vi "Dashboard Main.vi"() -> ()   [LabVIEW 2017]
uses:
  <vilib>/Rock Robotics/WPI/DriverStation/WPI_DriverStationAllianceInfo.ctl
  <vilib>/Utility/miscctls.llb/LVRowAndColumnTypeDef.ctl
  <vilib>/event_ctls.llb/eventvkey.ctl
  <vilib>/Rock Robotics/Network Tables/NT Read Numeric Array.vi
  <vilib>/Rock Robotics/WPI/Dashboard/WPI_DashboardLogging Global.vi
  <vilib>/Rock Robotics/Network Tables/NT Write Numeric Array.vi
  <vilib>/Rock Robotics/Network Tables/NT Write Boolean.vi
panel:
  in  "Camera Settings Right":T1={"Frame Rate"=30, "Compression"=30, "Size"=1, "DB Camera Config"=FALSE} {"Frame Rate" scale=1.0..30.0; "Compression" scale=100.0..-1.0; "Size" items=["640x480", "320x240", "160x120"]}
  in  "Camera Name Right":string(combo)="No Camera Selection"
  out "Camera Info":cluster{"Mbps LED":bool, "Mbps":dbl, "fps":dbl} {"fps" format="%#.1g"; "Mbps" format="%#.1g"}
  in  "Camera Settings":T1={"Frame Rate"=30, "Compression"=30, "Size"=1, "DB Camera Config"=FALSE} {"Frame Rate" scale=1.0..30.0; "Compression" scale=100.0..-1.0; "Size" items=["640x480", "320x240", "160x120"]}
  in  "TCP":refnum<k5>
  in  "Rec Mode":enum32{"Stop", "Record", "Playback"}(radio)
  out "Robot IP":string
  out "Image Message":string="Timeout in Camera Communications"
  in  "Dashboard Tab":T2(tab)=enum."Custom"
  in  "Select Auto":string(combo)="Select Autonomous ..."
  out "NT Connection":bool
  out "MotorChart R":cluster{"Numeric":dbl, "Numeric":dbl}(graph)
  out "MotorChart L":cluster{"Numeric":dbl, "Numeric":dbl}(graph)
  out "MotorSliders R":cluster{"MotorSlide1":dbl, "MotorSlide2":dbl} {"MotorSlide2" scale=-1.0..1.0 scale format="%#_2e"; "MotorSlide1" scale=-1.0..1.0 scale format="%#_2e"}
  out "MotorSliders L":cluster{"MotorSlide1":dbl, "MotorSlide2":dbl} {"MotorSlide2" scale=-1.0..1.0 scale format="%#_2e"; "MotorSlide1" scale=-1.0..1.0 scale format="%#_2e"}
  out "Gyro":dbl(knob) scale=0.0..360.0
  out "JS1 Z":dbl(slide) scale=-1.0..1.0 scale format="%#_2e"
  out "JS1 Graph":cluster{"X":dbl, "Y":dbl}[](graph)
  out "JS1 Buttons":T3
  out "JS2 Z":dbl(slide) scale=-1.0..1.0 scale format="%#_2e"
  out "JS2 Graph":cluster{"X":dbl, "Y":dbl}[](graph)
  out "JS2 Buttons":T3
  out "Mode":T4(ring)=enum."Auto Disabled"
  out "Camera Image Right":T5(plugin-control)
  in  "DB/String 9":string
  in  "DB/String 8":string
  in  "DB/String 7":string
  in  "DB/String 6":string
  in  "DB/String 5":string
  in  "DB/String 4":string
  in  "DB/String 3":string
  in  "DB/String 2":string
  in  "DB/String 1":string
  in  "DB/String 0":string
  in  "DB/Slider 0":dbl(slide) scale=0.0..5.0
  in  "DB/Slider 1":dbl(slide) scale=0.0..5.0
  in  "DB/Slider 2":dbl(slide) scale=0.0..5.0
  in  "DB/Slider 3":dbl(slide) scale=0.0..5.0
  out "DB/LED 3":bool
  out "DB/LED 2":bool
  out "DB/LED 1":bool
  out "DB/LED 0":bool
  in  "DB/Button 3":bool
  in  "DB/Button 2":bool
  in  "DB/Button 1":bool
  in  "DB/Button 0":bool caption="New Name"
  in  "Delay":dbl
  in  "NotPurePursuit":bool
  in  "Battery Number":string
  out "Opponent Left Switch":bool
  out "Opponent Right Switch":bool
  out "Center Left Scale":bool
  out "Center Right Scale":bool
  out "Our Left Team Switch":bool
  out "Our Right Team Switch":bool
  in  "Position":u32=3
  in  "Routine":u32
  in  "SwitchOtherClose":u32
  in  "SwitchOtherNotClose":u32
  in  "ScaleOtherClose":u32
  in  "ScaleOtherNotClose":u32
  in  "Test Slider":dbl(slide) scale=0.0..100.0 scale format="%#_3g"
  in  "On/Off":bool caption="Solenoid"
  in  "Test Name":u16(ring) items=["Select the test to run..."]
  in  "Test Tree":string(tree)
  in  "Motor":cluster{"Value":dbl, "Enable":bool} {"Value" scale=-1.0..1.0 scale format="%#_3g"}
  out "Progress":T6 {"Test Progress" scale=0.0..100.0}
  in  "Rev/Fwd":cluster{"Forward":bool, "Reverse":bool}
  in  "Test Ring":u16(ring) items=["Monochrome", "Color"]
  out "Cmd Status":string
  in  "Execute Command":bool
  in  "Command Params":string[][](table)
  in  "Command Selection":i32(listbox)
  in  "CheckList":i32(listbox)
  out "Tree":string(tree)
  out "Camera Image":T5(plugin-control)
  out "Background":bool
  in  "Camera Name":string(combo)="No Camera Selection"
  # "HW"
  # "HW"
  # "Joysticks"
  # "Drive Motors"
  # "Front"
  # "Right"
  # "Left"
  # "Back"
  # "0 - Definitely Switch\n1 - Definitely Scale\n2 -  Switch if in front, else scale\n3 - Scale if in front, else switch\n4 - Switch if in front, else cross line\n5 - Scale if in front, else cross line\n6 - Drive across line"
  # "TWO CUBE"
  # "Other one is close"
  # "Other one is not close"
  # "At Switch"
  # "0 - Nothing\n1 - Switch\n2 - Scale"
  # "(Seconds)"
  # "At Scale"
  # "1"
  # "2"
  # "3"
  # "4"
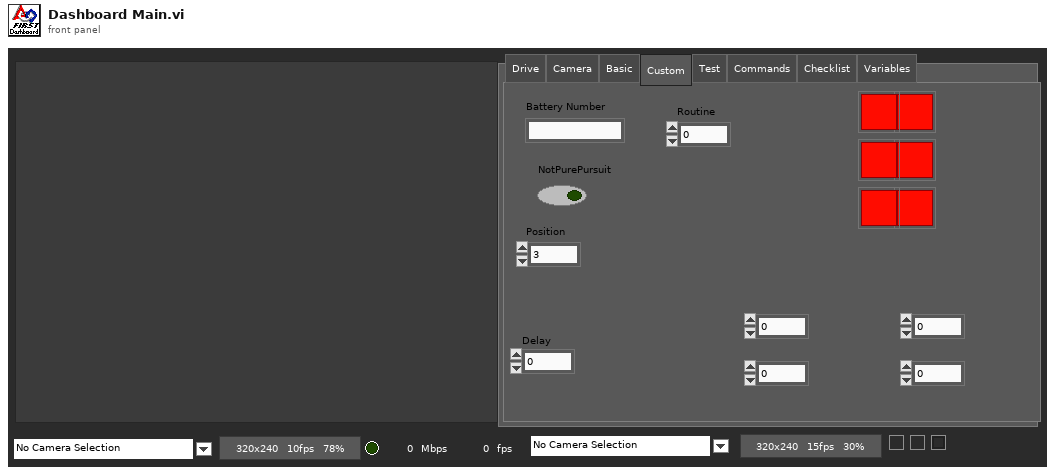
[diagram p1: front panel]
types:
  T1 = cluster{"Frame Rate":i32, "Compression":i32, "Size":u16, "DB Camera Config":bool}
  T2 = enum32{"Drive", "Camera", "Basic", "Custom", "Test", "Commands", "Checklist", "Variables"}
  T3 = cluster{bool, bool, bool, bool, bool, bool, bool, bool, bool, bool, bool, bool}
  T4 = enum8{"Tele-Op Disabled", "Tele-Op Enabled", "Auto Disabled", "Auto Enabled", "Test Disabled", "Test Enabled", "Disconnected", "No Code", "E-Stop"}
  T5 = typedef "IMAQ Image.ctl" = refnum<image>
  T6 = cluster{"Test Progress":u8, "Test Progress Text":string}
  T7 = cluster{"Save Path":path, "Interval (s)":dbl, "Keep":i32}
  T8 = typedef "Image Type" = u32
  T9 = cluster{"IDs":cluster{"RPC field ID":u16, "Unique ID":u16}, "String":string}
  T10 = cluster{"Error Strings":string, "Disable Counts":cluster{u16, u16}, "Rail Faults":cluster{u16, u16, u16}, "Robot IP":string, "DB Mode":u8, "Event Info":cluster{"Name":string, "Type":u8, "Number":u16, "Replay":u8}}
  T11 = cluster{"Storage":cluster{"Disk Free":u64, "RAM Block":u32, "RAM free":u32}, "CPU Utilization":cluster{"CPU % ISR":sgl, "CPU % Time Crit":sgl, "CPU % Timed Str":sgl, "CPU % High":sgl, "CPU % Above":sgl, "CPU % Normal":sgl, "CPU % Low":sgl}, "CAN":cluster{"% Bus Utilization":sgl, "Bus Off Cnt":u32, "TX_FIFO Full Cnt":u32, "Receive Error Cnt":u8, "Transmit Error Cnt":u8}, "HID":cluster{"HID Outputs":u32, "Rumble Low":u16, "Rumble High":u16}[]}
  T12 = cluster{"Status bits":cluster{"Test Mode":bool, "Autonomous":bool, "Enabled":bool, "Code Start":bool, "Brownout":bool, "Reserved 2":bool, "Reserved 3":bool, "E-Stop":bool}, "Code Trace":cluster{"Disabled":bool, "TeleOp":bool, "Auto":bool, "Test":bool}, "Controller Type":enum16{"unknown", "cRIO", "roboRio"}, "Code?":enum16{"unknown", "noCode", "code"}, "Battery V":dbl}
  T13 = cluster{"Control Bits":cluster{"TestMode":bool, "Autonomous":bool, "Enabled":bool, "FMS Present":bool, bool, bool, bool, "E-Stop":bool}, "Team Station ":u8, "Countdown":sgl, "Joystick Values":cluster{"Axes":dbl[], "Buttons":bool[], "POVs":i16[]}[]}
  T14 = cluster{"Axes":dbl[], "Buttons":bool[], "POVs":i16[]}[]
  T15 = cluster{"Axes":dbl[], "Buttons":bool[], "POVs":i16[]}
  T16 = cluster{"Buttons[0]":bool, "Buttons[1]":bool, "Buttons[2]":bool, "Buttons[3]":bool, "Buttons[4]":bool, "Buttons[5]":bool, "Buttons[6]":bool, "Buttons[7]":bool, "Buttons[8]":bool, "Buttons[9]":bool, "Buttons[10]":bool, "Buttons[11]":bool}
  T17 = cluster{"Camera Image":refnum<vi>, "Dashboard Tab":refnum<vi>, "Background":refnum<vi>, "Rec Mode":refnum<vi>, "Test Slider":refnum<vi>, "On/Off ":refnum<vi>, "Test Ring":refnum<vi>, "Rev/Fwd":refnum<vi>, "Test Name":refnum<vi>, "Motor":refnum<vi>, "Progress":refnum<vi>, "CheckList":refnum<vi>, "Tree":refnum<vi>, "Test Tree":refnum<vi>, "Command Params":refnum<vi>, "Command Selection":refnum<vi>, "Execute Command":refnum<vi>, "Cmd Status":refnum<vi>, "Camera Settings":refnum<vi>, "Camera Name":refnum<vi>, "Camera Info":refnum<vi>, "Camera Settings Right":refnum<vi>, "Camera Name Right":refnum<vi>, "Camera Image Right":refnum<vi>}
  T18 = cluster{"Camera Name":string, string, "Saved DB Images Info":cluster{"Save Path":path, "Interval (s)":dbl, "Keep":i32}}
  T19 = cluster{"Camera Name Right":string, string, "Saved DB Images Info":cluster{"Save Path":path, "Interval (s)":dbl, "Keep":i32}}
  T20 = typedef "WPI_DriverStationAllianceInfo.ctl" = enum16{"Red", "Blue", "Invalid"}
  T21 = cluster{"Operation":enum16{"Update", "Clear"}, "Color Box":u32}[]
  T22 = typedef "eventvkey.ctl" = enum16{"ASCII", "Enter", "Return", "Shift", "Ctrl", "Alt", "Cmd", "Opt", "Caps", "NumLock", "Clear", "Break", "Up", "Down", "Left", "Right", "Insert", "Delete", "Home", "End", "PageUp", "PageDown", "Escape", "Help", "Pause", "ScrollLock", "F1", "F2", "F3", "F4", "F5", "F6", "F7", "F8", "F9", "F10", "F11", "F12", "F13", "F14", "F15", "F16", "F17", "F18", "F19", "F20", "F21", "F22", "F23", "F24", "Play", "VolumeUp", "VolumeDown", "Mute", "Two Byte Char"}
  T23 = cluster{"Image Size":bool, "Image Type":bool, "Pixel Value":bool, "ROI Information":bool, "Zoom Factor":bool}
  T24 = cluster{"Operation":enum16{"Update", "Clear"}, "Color Box":u32}
  T25 = typedef "LVRowAndColumnTypeDef.ctl" = cluster{"Row":i32, "Column":i32}
  T26 = cluster{"Shift":bool, "Ctrl":bool, "Alt":bool, "Cmd":bool, "Opt":bool}
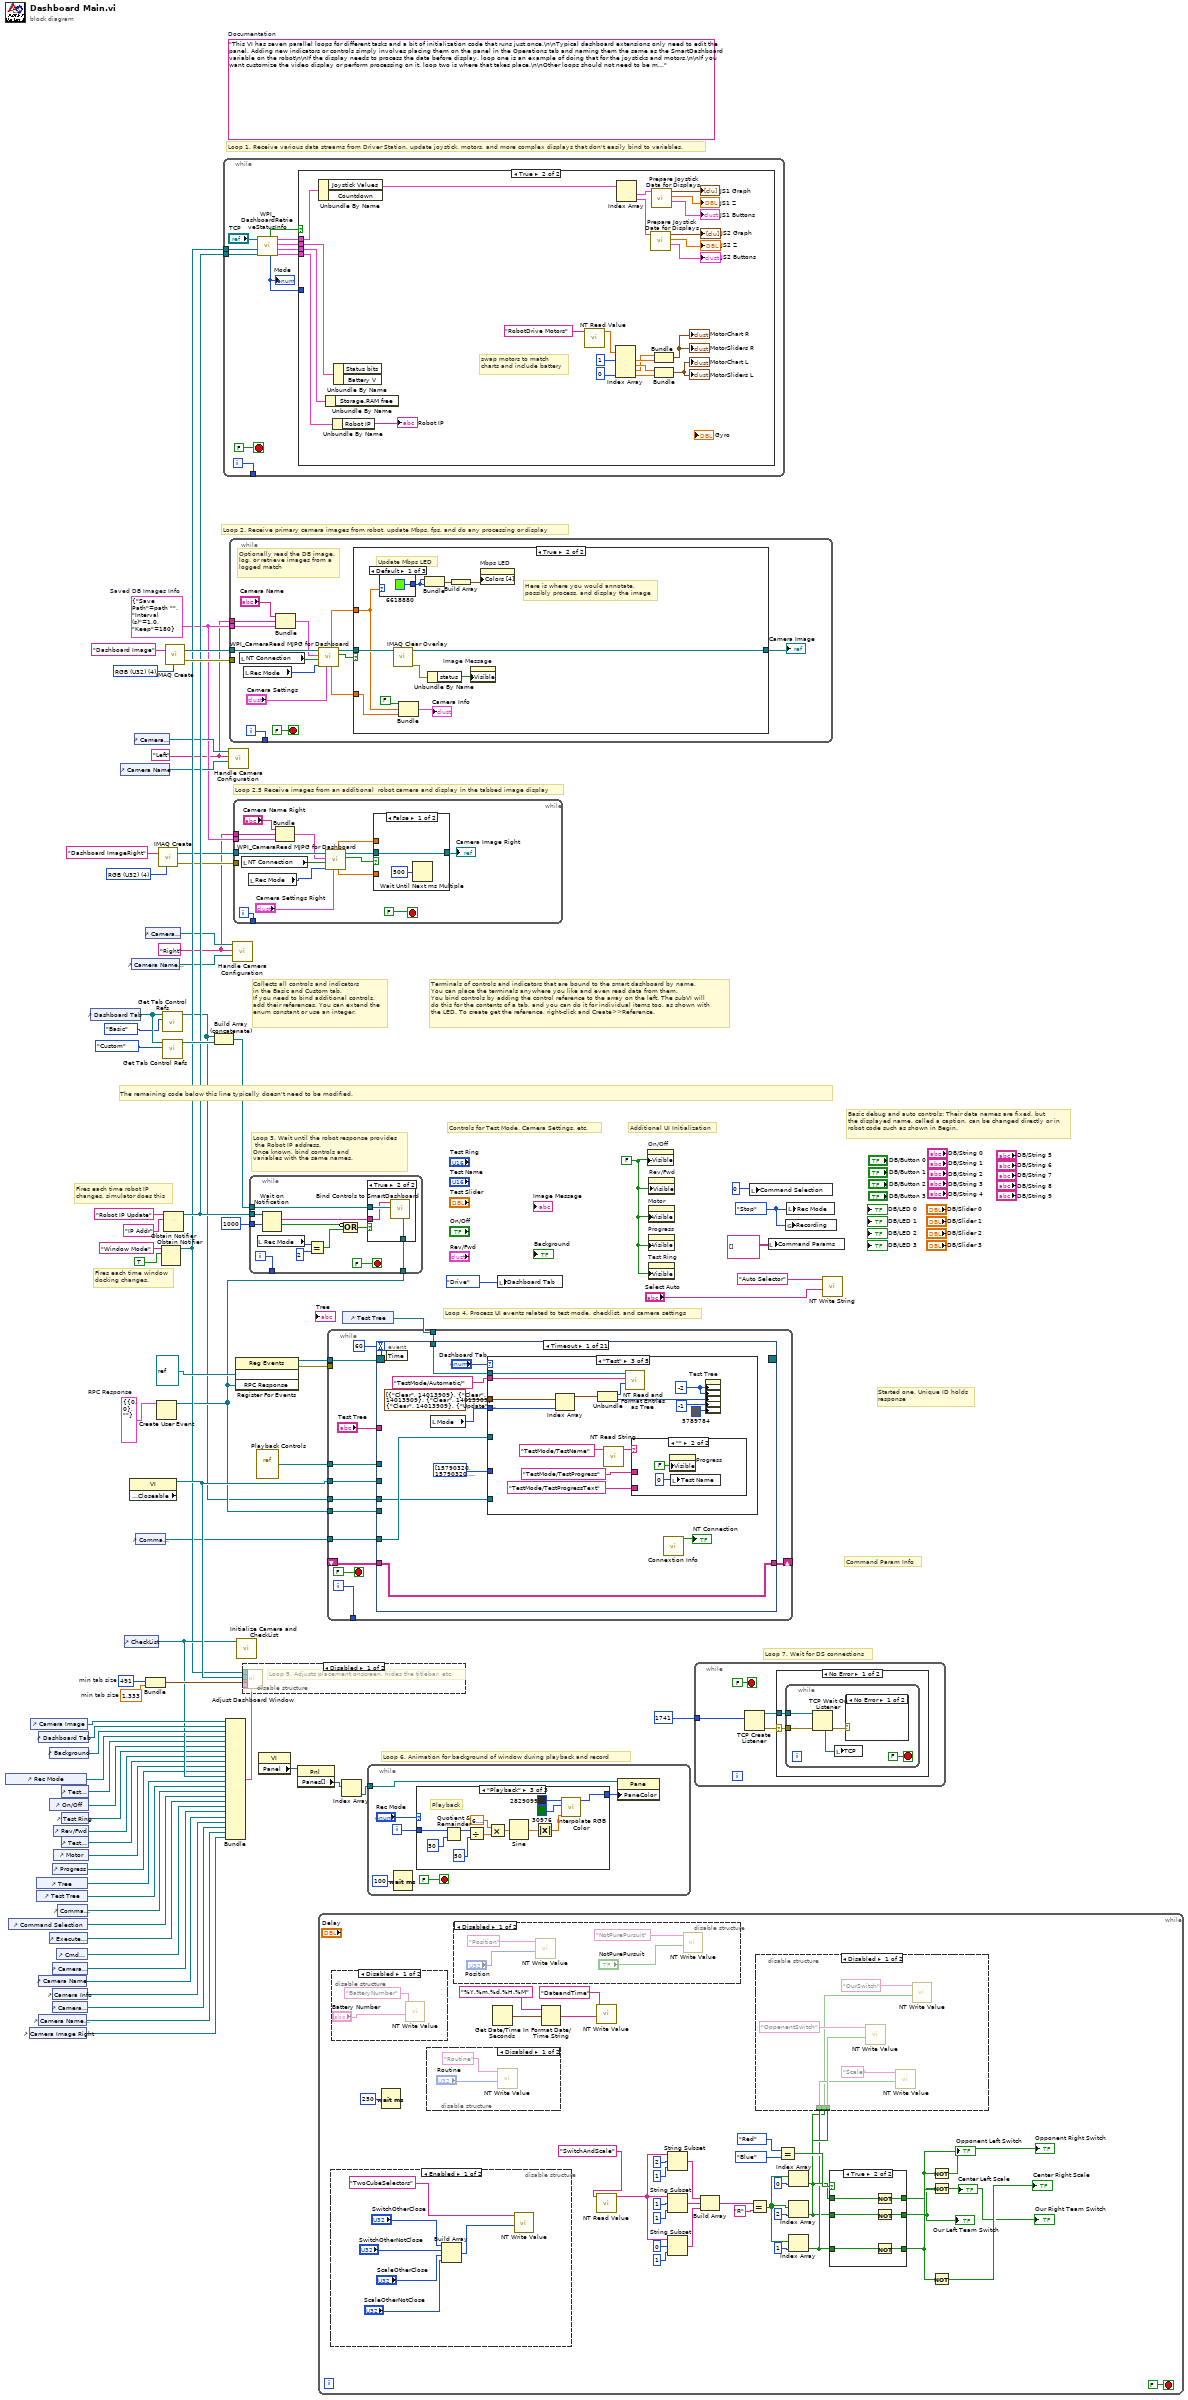
[diagram p0: block diagram]
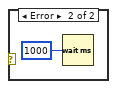
[diagram p10: hidden frame]
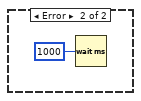
[diagram p11: hidden frame]
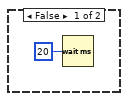
[diagram p12: hidden frame]
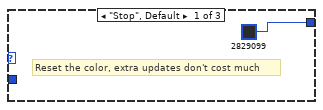
[diagram p13: hidden frame]
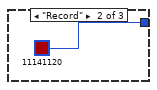
[diagram p14: hidden frame]
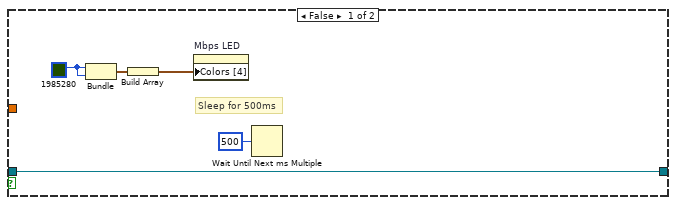
[diagram p16: hidden frame]
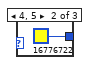
[diagram p17: hidden frame]
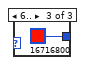
[diagram p18: hidden frame]
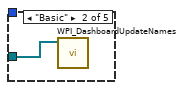
[diagram p20: hidden frame]
diagram:
  w3 = T7 {"Save Path"=path "", "Interval (s)"=1.0, "Keep"=180}  # Saved DB Images Info
  w2 = "Right"
  w1 = "Left"
  w13 = T8 4 items=["Grayscale (U8)", "Grayscale (I16)", "Grayscale (SGL)", "Complex (CSG)", "RGB (U32)", "HSL (U32)", "RGB (U64)"] ("Image Type")
  w29 = T9 {"IDs"={"RPC field ID"=0, "Unique ID"=0}, "String"=""}  # RPC Response
  w52 = 491  # min tab size
  w51 = 1.333  # min tab size
  w59 = enum32{"Stop", "Record", "Playback"}."Stop" ("Rec Mode")
  w36 = FALSE ("Visible")
  (unwired) "This VI has seven parallel loops for different tasks and a bit of initialization code that runs just once.\n\nTypical dashboard extensions only need to edit the panel. Adding new indicators or controls simply involves placing them on the panel in the Operations tab and naming them the same as the SmartDashboard variable on the robot\n\nIf the display needs to process the data before display, loop one is an example of doing that for the joysticks and motors.\n\nIf you want customize the video display or perform processing on it, loop two is where that takes place.\n\nOther loops should not need to be modified. They are pretty standard, and document the task they perform."  # Documentation
  w76 = T8 4 items=["Grayscale (U8)", "Grayscale (I16)", "Grayscale (SGL)", "Complex (CSG)", "RGB (U32)", "HSL (U32)", "RGB (U64)"] ("Image Type")
  # "Loop 2.5 Receive images from an additional  robot camera and display in the tabbed image display"
  # "Command Param Info"
  # "Started one, Unique ID holds\nresponse"
  # "Loop 7. Wait for DS connections"
  # "Basic debug and auto controls: Their data names are fixed, but\nthe displayed name, called a caption, can be changed directly or in\nrobot code such as shown in Begin."
  # "Controls for Test Mode, Camera Settings, etc."
  # "Additional UI Initialization"
  # "Loop 6. Animation for background of window during playback and record"
  # "Fires each time robot IP\nchanges, simulator does this"
  # "Fires each time window\ndocking changes."
  # "Collects all controls and indicators\nin the Basic and Custom tab.\nIf you need to bind additional controls,\nadd their references. You can extend the\nenum constant or use an integer."
  # "The remaining code below this line typically doesn't need to be modified."
  # "Loop 4. Process UI events related to test mode, checklist, and camera settings"
  # "Terminals of controls and indicators that are bound to the smart dashboard by name.\nYou can place the terminals anywhere you like and even read data from them.\nYou bind controls by adding the control reference to the array on the left. The subVI will\ndo this for the contents of a tab, and you can do it for individual items too, as shown with\nthe LED. To create get the reference, right-click and Create>>Reference."
  # "Loop 3. Wait until the robot response provides\n the Robot IP address.\nOnce known, bind controls and\nvariables with the same names."
  # "Loop 1. Receive various data streams from Driver Station, update joystick, motors, and more complex displays that don't easily bind to variables."
  # "Loop 2. Receive primary camera images from robot, update Mbps, fps, and do any processing or display"
  n1 = control-ref of="Rec Mode"() -> (w42:refnum<vi>)
  n2 = control-ref of="Command Selection"() -> (w28:refnum<vi>)
  n3 = control-ref of="Camera Image Right"() -> (w6:refnum<vi>)
  n4 = control-ref of="Camera Image"() -> (w54:refnum<vi>)
  n5 = control-ref of="Tree"() -> (w46:refnum<vi>)
  n6 = control-ref of="Test Tree"() -> (w45:refnum<vi>)
  n7 = control-ref of="Dashboard Tab"() -> (w53:refnum<vi>)
  n8 = control-ref of="Camera Name"() -> (w19:refnum<vi>)
  n9 = control-ref of="Camera Name Right"() -> (w7:refnum<vi>)
  n10 = control-ref of="Execute Command"() -> (w30:refnum<vi>)
  n11 = control-ref of="Background"() -> (w49:refnum<vi>)
  n12 = control-ref of="On/Off"() -> (w40:refnum<vi>)
  n13 = control-ref of="Progress"() -> (w37:refnum<vi>)
  n14 = control-ref of="Camera Settings"() -> (w20:refnum<vi>)
  n15 = control-ref of="Camera Info"() -> (w18:refnum<vi>)
  n16 = control-ref of="Camera Settings Right"() -> (w8:refnum<vi>)
  n17 = control-ref of="Rev/Fwd"() -> (w38:refnum<vi>)
  n18 = control-ref of="Motor"() -> (w43:refnum<vi>)
  n19 = control-ref of="Cmd Status"() -> (w24:refnum<vi>)
  n20 = control-ref of="Command Params"() -> (w31:refnum<vi>)
  n21 = control-ref of="Test Slider"() -> (w41:refnum<vi>)
  n22 = control-ref of="Test Ring"() -> (w39:refnum<vi>)
  n23 = control-ref of="Test Name"() -> (w44:refnum<vi>)
  n24 = control-ref of="Dashboard Tab"() -> (w57:refnum<vi>)
  n25 = control-ref of="Camera Name"() -> (w21:refnum<vi>)
  n26 = control-ref of="CheckList"() -> (w47:refnum<vi>)
  n27 = property class="VI" props=["Front Panel.Closeable"]() -> (reference out=w58:refnum<vi>)  [unwired: 2 in, 2 out]
  n28 = control-ref of="Camera Name Right"() -> (w9:refnum<vi>)
  n29 = control-ref of="Camera Settings"() -> (w22:refnum<vi>)
  n30 = control-ref of="Command Params"() -> (w23:refnum<vi>)
  n31 = control-ref of="Camera Settings Right"() -> (w10:refnum<vi>)
  n32 = Bundle("min tab size"=w52, "min tab size"=w51) -> (w50:cluster{"min tab size":i32, "min tab size":dbl})  [unwired: 1 in]
  n33 = Create User Event(user event datatype=w29) -> (user event=w25:refnum<user-event>)  [unwired: 1 in, 1 out]
  n34 = call "IMAQ Create"("Image Name"="Dashboard ImageRight", "Image Type"=w13) -> ("New Image"=w12:T5, "error out"=w11:errorcluster)  [unwired: 2 in, 1 out]
  n35 = Obtain Notifier(name (unnamed)="Window Mode", notification data type=TRUE) -> (notifier out=w34:refnum<notifier>)  [unwired: 2 in, 2 out]
  n36 = call <vilib>:"Get Tab Control Refs.vi"("Page Index"=T2."Basic" ("Dashboard Tab"), "TabControl in"=w57) -> ("ControlsOnPage"=w17:refnum<vi>[])  [unwired: 9 in]
  n37 = call <vilib>:"Get Tab Control Refs.vi"("Page Index"=T2."Custom" ("Dashboard Tab"), "TabControl in"=w57) -> ("ControlsOnPage"=w56:refnum<vi>[])  [unwired: 9 in]
  n38 = Obtain Notifier(name (unnamed)="Robot IP Update", notification data type="IP Addr" ("name (unnamed)")) -> (notifier out=w35:refnum<notifier>)  [unwired: 2 in, 2 out]
  n39 = call "IMAQ Create"("Image Name"="Dashboard Image", "Image Type"=w76) -> ("New Image"=w74:T5, "error out"=w73:errorcluster)  [unwired: 2 in, 1 out]
  n40 = Build Array (concatenate)(w17, w56) -> (w55:refnum<vi>[])
  n41 = while {
    tunnel: [w86] -> _
    tunnel: w35 -> [w80]
    tunnel: w34 -> [w77]
    i -> [w86]
    stop <- FALSE stop-if-true
    n42 = call <vilib>:"WPI_DashboardRetrieveStatusInfo.vi"("Binding Refnum"=w80, "Window Mode Notifier"=w77, "TCP Cnx"="TCP") -> ("Power and Errors"=w81:T10, "Robot Metrics"=w84:T11, "Status Info"=w85:T12, "Control Info"=w82:T13, "Robot Mode"=w79:T4, "Process?"=w83:bool)  [unwired: 3 in]
    "Mode" <- w79
    n43 = case shown="True" w83 {
      tunnel: w85 -> [_ w112]
      tunnel: w84 -> [_ w111]
      tunnel: w82 -> [_ w110]
      tunnel: w81 -> [_ w109]
      tunnel: w79 -> [_ _]
      frame False {
        n44 = Wait (ms)(milliseconds to wait=u32 20) -> ()  [unwired: 1 out]
      }
      frame True {
        # "swap motors to match\ncharts and include battery"
        n45 = Unbundle By Name(w110) -> ("Joystick Values"=w100:T14)  [unwired: 1 out]
        n46 = Unbundle By Name(w111) -> ()  [unwired: 1 out]
        n47 = Unbundle By Name(w109) -> ("Robot IP"=→"Robot IP":string)
        n48 = Unbundle By Name(w112) -> ()  [unwired: 2 out]
        n49 = call-poly <vilib>:"NT Read Value.vi"("Name"="RobotDrive Motors") -> ("Numeric Array"=w90:dbl[])  [unwired: 9 in, 1 out]
        n50 = Index Array(array=w90, index #1=1, index #4=0) -> (element #1=w104:dbl, element #2=w105:dbl, element #3=w103:dbl, element #4=w108:dbl)  [unwired: 2 in]
        n51 = Index Array(array=w100) -> (element #1=w99:T15, element #2=w95:T15)  [unwired: 2 in]
        n52 = call "Prepare Joystick Data for Displays.vi"("Joystick Values"=w95) -> ("Buttons"=→"JS2 Buttons":T16, "Z Axis"=→"JS2 Z":dbl, "Cartesian Data"=→"JS2 Graph":cluster{"X axis":dbl, "X axis":dbl}[])  [unwired: 8 in]
        n53 = call "Prepare Joystick Data for Displays.vi"("Joystick Values"=w99) -> ("Buttons"=→"JS1 Buttons":T16, "Z Axis"=→"JS1 Z":dbl, "Cartesian Data"=→"JS1 Graph":cluster{"X axis":dbl, "X axis":dbl}[])  [unwired: 8 in]
        n54 = Bundle("Numeric"=w103, "Numeric"=w104) -> (→"MotorChart R" →"MotorSliders R":cluster{"Numeric":dbl, "Numeric":dbl})  [unwired: 1 in]
        n55 = Bundle("Numeric"=w105, "Numeric"=w108) -> (→"MotorChart L" →"MotorSliders L":cluster{"Numeric":dbl, "Numeric":dbl})  [unwired: 1 in]
      }
    }
  }
  n56 = Bundle("Camera Image"=w54, "Dashboard Tab"=w53, "Background"=w49, "Rec Mode"=w42, "Test Slider"=w41, "On/Off"=w40, "Test Ring"=w39, "Rev/Fwd"=w38, "Test Name"=w44, "Motor"=w43, "Progress"=w37, "CheckList"=w47, "Tree"=w46, "Test Tree"=w45, "Command Params"=w31, "Command Selection"=w28, "Execute Command"=w30, "Cmd Status"=w24, "Camera Settings"=w20, "Camera Name"=w19, "Camera Info"=w18, "Camera Settings Right"=w8, "Camera Name Right"=w7, "Camera Image Right"=w6) -> (w48:T17)  [unwired: 1 in]
  n57 = call "Handle Camera Configuration.vi"("CameraNameRef"=w21, "Display Name"=w1, "ClusterRef"=w22) -> ()  [unwired: 9 in]
  n58 = while {
    tunnel: w74 -> [w125]
    tunnel: w73 -> [_]
    tunnel: [w126] -> _
    tunnel: w3 -> [w116]
    tunnel: w1 -> [w113]
    i -> [w126]
    stop <- FALSE stop-if-true
    # "Optionally read the DB image,\nlog, or retrieve images from a\nlogged match"
    n59 = local read "NT Connection"() -> (w117:bool)
    n60 = local read "Rec Mode"() -> (w121:enum32{"Stop", "Record", "Playback"})
    n61 = Bundle("Camera Name"="Camera Name", w113, "Saved DB Images Info"=w116) -> (w115:T18)  [unwired: 1 in]
    n62 = call <vilib>:"WPI_CameraRead MJPG for Dashboard.vi"("Camera Settings"="Camera Settings", "Rec Mode"=w121, "NT Connection"=w117, "Capture Info"=w115, "Refnum in"=w125) -> ("Active"=w123:bool, "Refnum out"=w124:T5, "FPS"=w122:dbl, "Bandwidth (Mbps)"=w120:dbl)  [unwired: 3 in]
    n63 = case shown="True" w123 {
      tunnel: w124 -> [w128 w139]
      tunnel: w120 -> [_ w136]
      tunnel: w122 -> [_ w137]
      tunnel: [w128 w133] -> w118
      frame False {
        w130 = u32 1985280 ("Color Box")
        # "Sleep for 500ms"
        n64 = Bundle("Color Box"=w130, "Color Box"=w130) -> (w131:cluster{"Color Box":u32, "Color Box":u32})  [unwired: 1 out]
        n65 = Build Array(w131) -> (w129:cluster{"Color Box":u32, "Color Box":u32}[])
        n66 = property on="Mbps LED" class="Bool (strict)"("Colors [4]"=w129) -> ()  [unwired: 2 in, 2 out]
        n67 = Wait Until Next ms Multiple(millisecond multiple=u32 500) -> ()  [unwired: 1 out]
      }
      frame True {
        # "Here is where you would annotate,\npossibly process, and display the image"
        # "Update Mbps LED"
        n68 = case shown="Default" w136 {
          tunnel: [u32 6618880 ("Color Box") u32 16776722 ("Color Box") u32 16716800 ("Color Box")] -> w140
          frame Default {
          }
          frame 4, 5 {
          }
          frame 6.. {
          }
        }
        n69 = call "IMAQ Clear Overlay"("Image"=w139) -> ("error out"=w142:errorcluster, "Image Out"=w133:T5)  [unwired: 2 in, 7 out]
        n70 = Bundle(FALSE, "Bandwidth (Mbps)"=w136, "FPS"=w137) -> (→"Camera Info":cluster{bool, "Bandwidth (Mbps)":dbl, "FPS":dbl})  [unwired: 1 in]
        n71 = Bundle("Color Box"=w140, "Color Box"=w140) -> (w141:cluster{"Color Box":u32, "Color Box":u32})  [unwired: 1 out]
        n72 = Unbundle By Name(w142) -> ("status"=w143:bool)
        n73 = Build Array(w141) -> (w138:cluster{"Color Box":u32, "Color Box":u32}[])
        n74 = property on="Image Message" class="Str"("Visible"=w143) -> ()  [unwired: 2 in, 2 out]
        n75 = property on="Mbps LED" class="Bool (strict)"("Colors [4]"=w138) -> ()  [unwired: 2 in, 2 out]
      }
    }
    "Camera Image" <- w118
  }
  n76 = call "Handle Camera Configuration.vi"("CameraNameRef"=w9, "Display Name"=w2, "ClusterRef"=w10) -> ()  [unwired: 9 in]
  n77 = while {
    tunnel: w12 -> [w161]
    tunnel: w11 -> [_]
    tunnel: [w156] -> _
    tunnel: w3 -> [w150]
    tunnel: w2 -> [w147]
    i -> [w156]
    stop <- FALSE stop-if-true
    n78 = local read "NT Connection"() -> (w151:bool)
    n79 = local read "Rec Mode"() -> (w160:enum32{"Stop", "Record", "Playback"})
    n80 = Bundle("Camera Name Right"="Camera Name Right", w147, "Saved DB Images Info"=w150) -> (w149:T19)  [unwired: 1 in]
    n81 = call <vilib>:"WPI_CameraRead MJPG for Dashboard.vi"("Camera Settings"="Camera Settings Right", "Rec Mode"=w160, "NT Connection"=w151, "Capture Info"=w149, "Refnum in"=w161) -> ("Active"=w155:bool, "Refnum out"=w158:T5, "FPS"=w153:dbl, "Bandwidth (Mbps)"=w154:dbl)  [unwired: 3 in]
    n82 = case shown="False" w155 {
      tunnel: w158 -> [w162 w164]
      tunnel: w154 -> [_ _]
      tunnel: w153 -> [_ _]
      tunnel: [w162 w164] -> w152
      frame False {
        n83 = Wait Until Next ms Multiple(millisecond multiple=u32 500) -> ()  [unwired: 1 out]
      }
      frame True {
      }
    }
    "Camera Image Right" <- w152
  }
  n84 = register-events(refnum<vi> refnum, w25) -> (reference out=w63:refnum<event-registration>, error out=w62:errorcluster)  [unwired: 2 in]
  n85 = call "Initialize Camera and CheckList.vi"("ListBox in"=w47) -> ()  [unwired: 11 in]
  n86 = disable-structure shown="Disabled" {
    disable-tunnel: w58 -> [w168 _]
    disable-tunnel: w50 -> [w167 _]
    disable-tunnel: w48 -> [w166 _]
    disable-tunnel: w34 -> [w165 _]
    frame Disabled {
      # "Loop 5. Adjusts placement onscreen, hides the titlebar, etc."
      n87 = call "Adjust Dashboard Window.vi"("Sizing Refnums"=w166, "Size Constraints"=w167, "VI"=w168, "WIn Mode"=w165) -> ()  [unwired: 8 in]
    }
    frame Enabled {
    }
  }
  n88 = while {
    tunnel: w55 -> [w180]
    tunnel: w35 -> [w178]
    tunnel: [w176] -> _
    tunnel: u32 1000 ("milliseconds to wait") -> [w175]
    tunnel: w25 -> [w169]
    i -> [w176]
    stop <- FALSE stop-if-true
    n89 = local read "Rec Mode"() -> (w171:enum32{"Stop", "Record", "Playback"})
    n90 = Wait on Notification(notifier=w178, timeout in ms (-1)=w175) -> (notification=w177:string, timed out?=w173:bool)  [unwired: 2 in, 2 out]
    n91 = Equal?(x=w171, y=u16 2 ("Rec Mode")) -> (x = y?=w172:bool)
    n92 = Compound Arithmetic op=OR(invert w173, w172) -> (w174:bool)
    n93 = case shown="True" w174 {
      tunnel: w180 -> [_ w183]
      tunnel: w177 -> [_ w182]
      tunnel: w169 -> [_ w181]
      frame False {
      }
      frame True {
        n94 = call <vilib>:"Bind Controls to SmartDashboard.vi"("RPC ref"=w181, "Bound Control Refs"=w183, "Server IP Address"=w182) -> ()  [unwired: 9 in]
      }
    }
  }
  n95 = vi-ref "Playback Controls.vi"() -> (w64:refnum<vi>)
  n96 = property class="VI"() -> ("Panel"=w66:refnum<vi>)  [unwired: 2 in, 2 out]
  n97 = property class="Pnl"(reference=w66) -> ("Panes[]"=w67:refnum<vi>[])  [unwired: 1 in, 2 out]
  n98 = while {
    stop <- FALSE stop-if-true
    n99 = disable-structure shown="Enabled" {
      frame Enabled {
        n100 = Build Array("SwitchOtherClose", "SwitchOtherNotClose", "ScaleOtherClose", "ScaleOtherNotClose") -> (w223:u32[])
        n101 = call-poly <vilib>:"NT Write Value.vi"("Numeric Array"=w223, "Name"="TwoCubeSelectors") -> ()  [unwired: 9 in, 1 out]
      }
      frame Disabled {
      }
    }
    n102 = disable-structure shown="Disabled" {
      frame Disabled {
        n103 = call-poly <vilib>:"NT Write Value.vi"("String"="Battery Number", "Name"="BatteryNumber") -> ()  [unwired: 9 in, 1 out]
      }
      frame Enabled {
      }
    }
    n104 = Wait (ms)(milliseconds to wait=u32 250) -> ()  [unwired: 1 out]
    n105 = disable-structure shown="Disabled" {
      frame Disabled {
        n106 = call-poly <vilib>:"NT Write Value.vi"("Numeric"="Routine", "Name"="Routine") -> ()  [unwired: 9 in, 1 out]
      }
      frame Enabled {
      }
    }
    n107 = disable-structure shown="Disabled" {
      frame Disabled {
        n108 = call-poly <vilib>:"NT Write Value.vi"("Numeric"="Position", "Name"="Position") -> ()  [unwired: 9 in, 1 out]
        n109 = call-poly <vilib>:"NT Write Value.vi"("Boolean"="NotPurePursuit", "Name"="NotPurePursuit") -> ()  [unwired: 9 in, 1 out]
      }
      frame Enabled {
      }
    }
    n110 = Get Date/Time In Seconds() -> (seconds since 1Jan1904=w214:timestamp)
    n111 = Format Date/Time String(time format string (%c)="%Y.%m.%d.%H.%M", seconds (now)=w214) -> (date/time string=w213:string)  [unwired: 1 in]
    n112 = call-poly <vilib>:"NT Write Value.vi"("String"=w213, "Name"="DateandTime") -> ()  [unwired: 9 in, 1 out]
    n113 = call-poly <vilib>:"NT Read Value.vi"("Name"="SwitchAndScale") -> ("String"=w185:string)  [unwired: 9 in, 1 out]
    n114 = String Subset(string=w185, offset (0)=2, length (rest)=1 ("length (rest)")) -> (substring=w207:string)
    n115 = String Subset(string=w185, offset (0)=1, length (rest)=1 ("length (rest)")) -> (substring=w206:string)
    n116 = String Subset(string=w185, offset (0)=0, length (rest)=1 ("length (rest)")) -> (substring=w205:string)
    n117 = Build Array(w207, w206, w205) -> (w204:string[])
    n118 = Equal?(x=w204, y="R") -> (x = y?=w199:bool[])
    n119 = Equal?(x=WPI_DriverStationAllianceInfo."Red" ("y"), y=WPI_DriverStationAllianceInfo."Blue") -> (x = y?=w195:bool)
    n120 = Index Array(array=w199, index=0) -> (element=w188:bool)
    n121 = Index Array(array=w199, index=2) -> (element=w186:bool)
    n122 = Index Array(array=w199, index=1) -> (element=w187:bool)
    n123 = disable-structure shown="Disabled" {
      disable-tunnel: w188 -> [w235 _]
      disable-tunnel: w187 -> [w234 _]
      disable-tunnel: w186 -> [w233 _]
      frame Disabled {
        n124 = call-poly <vilib>:"NT Write Value.vi"("Boolean"=w235, "Name"="OppenentSwitch") -> ()  [unwired: 9 in, 1 out]
        n125 = call-poly <vilib>:"NT Write Value.vi"("Boolean"=w234, "Name"="Scale") -> ()  [unwired: 9 in, 1 out]
        n126 = call-poly <vilib>:"NT Write Value.vi"("Boolean"=w233, "Name"="OurSwitch") -> ()  [unwired: 9 in, 1 out]
      }
      frame Enabled {
      }
    }
    n127 = case shown="True" w195 {
      tunnel: w186 -> [w239 w243]
      tunnel: [w239 w242] -> w190
      tunnel: w187 -> [w241 w245]
      tunnel: [w241 w244] -> w193
      tunnel: w188 -> [w240 w247]
      tunnel: [w240 w246] -> w191
      frame False {
      }
      frame True {
        n128 = Not(x=w247) -> (.not. x?=w246:bool)
        n129 = Not(x=w243) -> (.not. x?=w242:bool)
        n130 = Not(x=w245) -> (.not. x?=w244:bool)
      }
    }
    "Opponent Left Switch" <- w191
    "Center Left Scale" <- w193
    "Our Left Team Switch" <- w190
    n131 = Not(x=w191) -> (.not. x?=→"Opponent Right Switch":bool)
    n132 = Not(x=w190) -> (.not. x?=→"Our Right Team Switch":bool)
    n133 = Not(x=w193) -> (.not. x?=→"Center Right Scale":bool)
  }
  n134 = Index Array(array=w67) -> (element=w65:refnum<vi>)  [unwired: 1 in]
  n135 = control-ref of="Test Tree"() -> (w68:refnum<vi>)
  n136 = while {
    tunnel: [w257] -> _
    tunnel: w68 -> [w256]
    tunnel: w64 -> [w255]
    tunnel: w63 -> [w254]
    tunnel: w62 -> [_]
    tunnel: w58 -> [w253]
    tunnel: w25 -> [w252]
    tunnel: w23 -> [w251]
    shift-right: [w250] -> _
    shift-left: _ -> [w249]
    tunnel: w17 -> [w248]
    i -> [w257]
    stop <- FALSE stop-if-true
    n137 = event shown="[0] Timeout" {
      selector: w254 -> [_ _ _ _ _ _ _ _ _ _ _ _ _ _ _ _ _ _ _ _ _]
      dyn-events: [_ _ _ _ _ _ _ _ _ _ _ _ _ _ _ _ w517 _ _ _ _] -> _
      timeout: u32 60 ("milliseconds to wait") -> [_ _ _ _ _ _ _ _ _ _ _ _ _ _ _ _ _ _ _ _ _]
      tunnel: w256 -> [w269 _ _ _ _ _ _ _ _ _ _ _ _ _ _ _ _ _ _ _ _]
      tunnel: "Test Tree" -> [_ _ _ _ _ _ _ _ _ _ _ w484 w492 w494 w498 w506 _ _ _ _ _]
      tunnel: w255 -> [_ _ _ _ _ _ _ _ _ _ _ _ _ _ _ _ w519 _ w537 _ _]
      tunnel: w253 -> [_ _ _ _ _ _ _ _ _ _ _ _ _ _ _ _ w515 _ _ _ _]
      tunnel: w252 -> [_ _ _ _ _ _ _ _ _ _ _ _ _ _ _ _ w513 _ _ _ _]
      tunnel: w251 -> [w264 _ _ _ _ _ w435 _ _ _ _ _ _ _ _ _ _ _ _ _ _]
      tunnel: [w263 w312 w414 w419 w428 w432 w433 w442 w452 w459 w471 w483 w490 w493 w497 w505 w512 w532 w534 w538 w551] -> w250
      tunnel: w249 -> [w263 w312 w414 w419 w428 w432 w433 _ _ w459 w471 w483 w490 w493 w497 w505 w512 w532 w534 w538 w551]
      tunnel: w248 -> [w261 _ _ _ _ _ _ _ _ _ _ _ _ _ _ _ _ _ _ _ _]
      event Timeout {
        n138 = event-data() -> ()  [unwired: 1 in, 1 out]
        n139 = local read "Mode"() -> (w266:T4)
        n140 = case shown="\"Test\"" "Dashboard Tab" {
          tunnel: w269 -> [_ _ w285 _ _]
          tunnel: "TestMode/Automatic/" ("Name Pattern") -> [_ _ w284 _ _]
          tunnel: T21 [{"Operation"=enum."Clear", "Color Box"=14013909}, {"Operation"=enum."Clear", "Color Box"=14013909}, {"Operation"=enum."Clear", "Color Box"=14013909}, {"Operation"=enum."Clear", "Color Box"=14013909}, {"Operation"=enum."Update", "Color Box"=14013909}, {"Operation"=enum."Update", "Color Box"=16777215}, {"Operation"=enum."Clear", "Color Box"=14013909}, {"Operation"=enum."Clear", "Color Box"=14013909}, {"Operation"=enum."Clear", "Color Box"=14013909}] -> [_ _ w277 _ w305]
          tunnel: w266 -> [_ _ w276 _ w304]
          tunnel: u32[] [15790320, 15790320, 15790320, 15790320, 16777215, 16777215, 15790320, 15790320, 15790320] -> [_ _ _ _ w310]
          tunnel: w264 -> [_ _ _ _ w298]
          tunnel: w261 -> [_ w271 _ _ _]
          frame "Custom", Default {
          }
          frame "Basic" {
            n141 = call <vilib>:"WPI_DashboardUpdateNames.vi"("Controls on Tab"=w271) -> ()  [unwired: 11 in]
          }
          frame "Test" {
            w283 = -2 ("Active Item:Row Number")
            n142 = Index Array(array=w277, index=w276) -> (element=w278:T24)
            n143 = Unbundle(w278) -> ("Operation"=w279:enum16{"Update", "Clear"}, "Color Box"=w280:u32)
            n144 = call <vilib>:"NT Read String.vi"("Name"="TestMode/TestName") -> ("String"=w274:string)  [unwired: 9 in, 1 out]
            n145 = call <vilib>:"NT Read and Format Entries as Tree.vi"("Operation"=w279, "Name Pattern"=w284, "Tree Refnum"=w285) -> ()  [unwired: 7 in, 2 out]
            n146 = case shown="\"\"" w274 {
              tunnel: "TestMode/TestProgress" ("Name") -> [w287 _]
              tunnel: "TestMode/TestProgressText" ("Name") -> [w286 _]
              frame Default {
                n147 = call <vilib>:"NT Read Number.vi"("Name"=w287) -> ("Numeric"=w288:dbl)  [unwired: 9 in, 1 out]
                n148 = call <vilib>:"NT Read String.vi"("Name"=w286) -> ("String"=w289:string)  [unwired: 9 in, 1 out]
                n149 = Bundle("Numeric"=w288, "String"=w289) -> (→"Progress":cluster{"Numeric":dbl, "String":string})  [unwired: 1 in]
              }
              frame "" {
                n150 = property on="Progress" class="Clust (strict)"("Visible"=FALSE) -> ()  [unwired: 2 in, 2 out]
                n151 = local write "Test Name"(u16 0) -> ()
              }
            }
            n152 = property on="Test Tree" class="Tree (strict)"("Active Item Row Number"=w283, "ActiveColNum"=w283, "CellBG"=w280, "Active Item Row Number"=-1 ("Active Item:Row Number"), "CellBG"=u32 5789784 ("Color Box")) -> ()  [unwired: 2 in, 2 out]
          }
          frame "Variables" {
            w295 = string[] ["CameraPublisher", "Usage", "DB"]  # Items to initially close
            n153 = First Call?() -> (First Call?: T/F=w296:bool)
            n154 = control-ref of="Tree"() -> (w297:refnum<vi>)
            n155 = Select(t=w295, s=w296, f=string[] []) -> (s? t:f=w293:string[])
            n156 = call <vilib>:"NT Read and Format Entries as Tree.vi"("Tags to  Close"=w293, "Tree Refnum"=w297) -> ()  [unwired: 8 in, 2 out]
          }
          frame "Commands" {
            w306 = u32 5789784 ("Color Box")
            w307 = T25 {"Row"=-1, "Column"=-2} ("Active Cell:Active Cell")
            w309 = T25 {"Row"=-2, "Column"=-2} ("Active Cell:Active Cell")
            n157 = Index Array(array=w310, index=w304) -> (element=w308:u32)
            n158 = Index Array(array=w305, index=w304) -> (element=w303:T24)
            n159 = Unbundle(w303) -> ("Operation"=w302:enum16{"Update", "Clear"})  [unwired: 1 out]
            n160 = local read "Command Selection"() -> (w301:i32)
            n161 = property on="Command Selection" class="MCListbox (strict)"("ActiveCell"=w309, "CellBG"=w308, "ActiveCell"=w307, "CellBG"=w306) -> ()  [unwired: 2 in, 2 out]
            n162 = call <vilib>:"WPI_DashboardUpdate RPC Info.vi"("Operation"=w302) -> ("update"=w300:bool, "commands"=w299:string[][])  [unwired: 9 in]
            n163 = property on="Command Selection" class="MCListbox (strict)"("ItemNames"=w299) -> ()  [unwired: 2 in, 2 out]
            n164 = property on="Command Params" class="Tbl (strict)"("Active Cell"=w309, "Cell BG Color"=w308, "Active Cell"=w307, "Cell BG Color"=w306) -> ()  [unwired: 2 in, 2 out]
            n165 = call <vilib>:"WPI_DashboardUpdate Command Params.vi"("Update"=w300, "NewVal"=w301, "Commands"=w299, "Param Tbl"=w298) -> ()  [unwired: 7 in, 1 out]
          }
        }
        n166 = call <vilib>:"Connextion Info.vi"() -> ("Connected"=→"NT Connection":bool)  [unwired: 10 in, 1 out]
      }
      event "Test Tree": Value Change {
        # "Show appropriate\ncontrols"
        n167 = event-data() -> ("CtlRef"=w315:refnum<vi>, "NewVal"=w313:string)  [unwired: 1 in]
        n168 = call <vilib>:"WPI_UtilitiesGetTreeIOName.vi"("NewVal"=w313, "TreeControl in"=w315) -> ("I/O Name"=w316:string)  [unwired: 9 in]
        n169 = case shown="\"Camera\"" w316 {
          selector: w316 -> [_ w323 _ w345 w354 _]
          tunnel: w313 -> [_ _ w342 w344 _ w361]
          tunnel: cluster{string[]}[] [{["640x480", "320x240", "160x120"]}, {["Auto", "Fixed indoor", "Fixed outdoor 1", "Fixed outdoor 2", "Fixed fluorescent 1", "Fixed fluorescent 2", "Hold current"]}, {["Auto", "Flicker-free 50 Hz", "Flicker-free 60 Hz", "Hold current"]}, {["None", "Prioritize frame rate", "Prioritize image quality"]}, {["Monochrome", "Color"]}] -> [_ _ _ _ _ w360]
          frame Default {
            w318 = FALSE ("Visible")
            w317 = FALSE ("Visible")
            n170 = property on="Motor" class="Clust (strict)"("Visible"=w317) -> ()  [unwired: 2 in, 2 out]
            n171 = property on="Test Ring" class="Ring (strict)"("Visible"=w317) -> ()  [unwired: 2 in, 2 out]
            n172 = property on="Rev/Fwd" class="Clust (strict)"("Visible"=w318) -> ()  [unwired: 2 in, 2 out]
            n173 = property on="On/Off" class="Bool (strict)"("Visible"=w318) -> ()  [unwired: 2 in, 2 out]
            n174 = property on="Test Slider" class="Slide (strict)"("Visible"=w318) -> ()  [unwired: 2 in, 2 out]
          }
          frame "Analog Out", "Motor", "PWM" {
            w324 = FALSE ("Visible")
            n175 = case shown="\"Analog Out\"" w323 {
              tunnel: [1.0 ("Value") -1.0 ("Value") 0.0 ("Value")] -> w322
              tunnel: [255.0 ("Value") 1.0 ("Value") 5.0 ("Value")] -> w321
              tunnel: [128.0 ("Value") 0.0 ("Value") 0.0 ("Value")] -> w320
              tunnel: [64.0 ("Value") 0.5 ("Value") 1.0 ("Value")] -> w319
              frame "PWM" {
              }
              frame "Motor", Default {
              }
              frame "Analog Out" {
              }
            }
            n176 = property on="Motor" class="Clust (strict)"("Visible"=TRUE) -> ()  [unwired: 2 in, 2 out]
            n177 = property on="Value" class="Slide (strict)"("Value"=w320, "Scale.Minimum"=w322, "Scale.Maximum"=w321, "Scale.Increment"=w319) -> ()  [unwired: 2 in, 2 out]
            n178 = property on="On/Off" class="Bool (strict)"("Visible"=w324) -> ()  [unwired: 2 in, 2 out]
            n179 = property on="Test Slider" class="Slide (strict)"("Visible"=w324) -> ()  [unwired: 2 in, 2 out]
            n180 = property on="Test Ring" class="Ring (strict)"("Visible"=w324) -> ()  [unwired: 2 in, 2 out]
            n181 = property on="Rev/Fwd" class="Clust (strict)"("Visible"=w324) -> ()  [unwired: 2 in, 2 out]
          }
          frame "Servo" {
            w340 = FALSE ("Visible")
            n182 = call <vilib>:"NT Read Number.vi"("Name"=w342) -> ("Numeric"=w341:dbl)  [unwired: 9 in, 1 out]
            n183 = property on="Test Slider" class="Slide (strict)"("Visible"=TRUE, "Scale.Maximum"=170.0 ("Scale.Range:Maximum")) -> ()  [unwired: 2 in, 2 out]
            n184 = local write "Test Slider"(w341) -> ()
            n185 = property on="Motor" class="Clust (strict)"("Visible"=w340) -> ()  [unwired: 2 in, 2 out]
            n186 = property on="Rev/Fwd" class="Clust (strict)"("Visible"=w340) -> ()  [unwired: 2 in, 2 out]
            n187 = property on="On/Off" class="Bool (strict)"("Visible"=w340) -> ()  [unwired: 2 in, 2 out]
            n188 = property on="Test Ring" class="Ring (strict)"("Visible"=w340) -> ()  [unwired: 2 in, 2 out]
          }
          frame "Relay", "Solenoid" {
            w343 = FALSE ("Visible")
            n189 = property on="Motor" class="Clust (strict)"("Visible"=w343) -> ()  [unwired: 2 in, 2 out]
            n190 = property on="Test Slider" class="Slide (strict)"("Visible"=w343) -> ()  [unwired: 2 in, 2 out]
            n191 = Search and Replace String(input string=w344, search string="/Value  **", replace string="/Direction") -> (result string=w350:string)  [unwired: 5 in, 3 out]
            n192 = property on="Test Ring" class="Ring (strict)"("Visible"=w343) -> ()  [unwired: 2 in, 2 out]
            n193 = call <vilib>:"NT Read String.vi"("Name"=w350) -> ("String"=w348:string)  [unwired: 9 in, 1 out]
            n194 = Equal?(x="Both directions", y=w348) -> (x = y?=w346:bool)
            n195 = Not(x=w346) -> (.not. x?=w347:bool)
            n196 = property on="Rev/Fwd" class="Clust (strict)"("Visible"=w346) -> ()  [unwired: 2 in, 2 out]
            n197 = property on="On/Off" class="Bool (strict)"("Visible"=w347, "Caption.Text"=w345) -> ()  [unwired: 2 in, 2 out]
          }
          frame "Compressor", "Digital Out" {
            w353 = FALSE ("Visible")
            # "Get direction and finish"
            n198 = property on="Motor" class="Clust (strict)"("Visible"=w353) -> ()  [unwired: 2 in, 2 out]
            n199 = property on="Test Slider" class="Slide (strict)"("Visible"=w353) -> ()  [unwired: 2 in, 2 out]
            n200 = property on="Test Ring" class="Ring (strict)"("Visible"=w353) -> ()  [unwired: 2 in, 2 out]
            n201 = property on="On/Off" class="Bool (strict)"("Visible"=TRUE, "Caption.Text"=w354) -> ()  [unwired: 2 in, 2 out]
            n202 = property on="Rev/Fwd" class="Clust (strict)"("Visible"=FALSE) -> ()  [unwired: 2 in, 2 out]
          }
          frame "Camera" {
            n203 = call <vilib>:"Get Last Path Segment.vi"("String in"=w361) -> ("String out"=w362:string)  [unwired: 10 in]
            n204 = property on="On/Off" class="Bool (strict)"("Visible"=FALSE) -> ()  [unwired: 2 in, 2 out]
            n205 = property on="Motor" class="Clust (strict)"("Visible"=FALSE) -> ()  [unwired: 2 in, 2 out]
            n206 = property on="Rev/Fwd" class="Clust (strict)"("Visible"=FALSE) -> ()  [unwired: 2 in, 2 out]
            n207 = case shown="\"White Balance  **\"" w362 {
              tunnel: w361 -> [w368 w377 w386 w395 w404 _ w410]
              tunnel: w360 -> [w366 w374 w383 w392 w401 _ _]
              frame "Size  **" {
                n208 = Index Array(array=w366) -> (element=w365:cluster{string[]})  [unwired: 1 in]
                n209 = call <vilib>:"NT Read String.vi"("Name"=w368) -> ("String"=w367:string)  [unwired: 9 in, 1 out]
                n210 = Unbundle(w365) -> (w363:string[])
                n211 = Match First String(2:w363, 3:w367) -> (0:w364:i32)  [unwired: 1 out]
                n212 = property on="Test Ring" class="Ring (strict)"("Value"=w364, "Strings []"=w363) -> ()  [unwired: 2 in, 2 out]
                n213 = property on="Test Ring" class="Ring (strict)"("Visible"=TRUE) -> ()  [unwired: 2 in, 2 out]
                n214 = property on="Test Slider" class="Slide (strict)"("Visible"=FALSE) -> ()  [unwired: 2 in, 2 out]
              }
              frame "White Balance  **" {
                n215 = Index Array(array=w374, index=1) -> (element=w375:cluster{string[]})
                n216 = call <vilib>:"NT Read String.vi"("Name"=w377) -> ("String"=w376:string)  [unwired: 9 in, 1 out]
                n217 = Unbundle(w375) -> (w372:string[])
                n218 = Match First String(2:w372, 3:w376) -> (0:w371:i32)  [unwired: 1 out]
                n219 = property on="Test Ring" class="Ring (strict)"("Value"=w371, "Strings []"=w372) -> ()  [unwired: 2 in, 2 out]
                n220 = property on="Test Ring" class="Ring (strict)"("Visible"=TRUE) -> ()  [unwired: 2 in, 2 out]
                n221 = property on="Test Slider" class="Slide (strict)"("Visible"=FALSE) -> ()  [unwired: 2 in, 2 out]
              }
              frame "Exposure  **" {
                n222 = Index Array(array=w383, index=2) -> (element=w384:cluster{string[]})
                n223 = call <vilib>:"NT Read String.vi"("Name"=w386) -> ("String"=w385:string)  [unwired: 9 in, 1 out]
                n224 = Unbundle(w384) -> (w380:string[])
                n225 = Match First String(2:w380, 3:w385) -> (0:w381:i32)  [unwired: 1 out]
                n226 = property on="Test Ring" class="Ring (strict)"("Value"=w381, "Strings []"=w380) -> ()  [unwired: 2 in, 2 out]
                n227 = property on="Test Ring" class="Ring (strict)"("Visible"=TRUE) -> ()  [unwired: 2 in, 2 out]
                n228 = property on="Test Slider" class="Slide (strict)"("Visible"=FALSE) -> ()  [unwired: 2 in, 2 out]
              }
              frame "Exposure Priority  **" {
                n229 = Index Array(array=w392, index=3) -> (element=w393:cluster{string[]})
                n230 = call <vilib>:"NT Read String.vi"("Name"=w395) -> ("String"=w394:string)  [unwired: 9 in, 1 out]
                n231 = Unbundle(w393) -> (w389:string[])
                n232 = Match First String(2:w389, 3:w394) -> (0:w390:i32)  [unwired: 1 out]
                n233 = property on="Test Ring" class="Ring (strict)"("Value"=w390, "Strings []"=w389) -> ()  [unwired: 2 in, 2 out]
                n234 = property on="Test Ring" class="Ring (strict)"("Visible"=TRUE) -> ()  [unwired: 2 in, 2 out]
                n235 = property on="Test Slider" class="Slide (strict)"("Visible"=FALSE) -> ()  [unwired: 2 in, 2 out]
              }
              frame "Color Enable  **" {
                n236 = Index Array(array=w401, index=4) -> (element=w402:cluster{string[]})
                n237 = call <vilib>:"NT Read String.vi"("Name"=w404) -> ("String"=w403:string)  [unwired: 9 in, 1 out]
                n238 = Unbundle(w402) -> (w398:string[])
                n239 = Match First String(2:w398, 3:w403) -> (0:w399:i32)  [unwired: 1 out]
                n240 = property on="Test Ring" class="Ring (strict)"("Value"=w399, "Strings []"=w398) -> ()  [unwired: 2 in, 2 out]
                n241 = property on="Test Ring" class="Ring (strict)"("Visible"=TRUE) -> ()  [unwired: 2 in, 2 out]
                n242 = property on="Test Slider" class="Slide (strict)"("Visible"=FALSE) -> ()  [unwired: 2 in, 2 out]
              }
              frame Default {
                n243 = property on="Test Ring" class="Ring (strict)"("Visible"=FALSE) -> ()  [unwired: 2 in, 2 out]
                n244 = property on="Test Slider" class="Slide (strict)"("Visible"=FALSE) -> ()  [unwired: 2 in, 2 out]
              }
              frame "Brightness  **", "Color Level  **", "Compression  **", "FPS  **", "Sharpness  **" {
                n245 = call <vilib>:"NT Read Number.vi"("Name"=w410) -> ("Numeric"=w409:dbl)  [unwired: 9 in, 1 out]
                n246 = local write "Test Slider"(w409) -> ()
                n247 = property on="Test Slider" class="Slide (strict)"("Visible"=TRUE, "Scale.Maximum"=100.0 ("Scale.Range:Maximum")) -> ()  [unwired: 2 in, 2 out]
                n248 = property on="Test Ring" class="Ring (strict)"("Visible"=FALSE) -> ()  [unwired: 2 in, 2 out]
              }
            }
          }
        }
        n249 = property on="Progress" class="Clust (strict)"("Visible"=FALSE) -> ()  [unwired: 2 in, 2 out]
      }
      event "Test Name": Mouse Enter {
        # "Populate the ring with the list of tests"
        n250 = event-data() -> ()  [unwired: 1 in, 1 out]
        n251 = call <vilib>:"NT Read String Array.vi"("Name"="TestMode/TestList") -> ("String Array"=w418:string[])  [unwired: 9 in, 1 out]
        n252 = Build Array (concatenate)("Select the test to run...", w418) -> (w417:string[])
        n253 = property on="Test Name" class="Ring (strict)"("Strings []"=w417) -> ()  [unwired: 2 in, 2 out]
      }
      event "Test Name": Value Change {
        w420 = FALSE ("Visible")
        # "Tell the robot the test name to run"
        n254 = event-data() -> ("NewVal"=w424:u16)  [unwired: 1 in]
        n255 = property on="Test Name" class="Ring (strict)"() -> ("Strings []"=w425:string[])  [unwired: 2 in, 2 out]
        n256 = local write "Progress"(T6 {"Test Progress"=0, "Test Progress Text"=""} ("Progress")) -> ()
        n257 = Index Array(array=w425, index=w424) -> (element=w423:string)
        n258 = call <vilib>:"NT Write String.vi"("String"=w423, "Name"="TestMode/TestName") -> ()  [unwired: 9 in, 1 out]
        n259 = property on="Progress" class="Clust (strict)"("Visible"=TRUE) -> ()  [unwired: 2 in, 2 out]
        n260 = property on="Motor" class="Clust (strict)"("Visible"=w420) -> ()  [unwired: 2 in, 2 out]
        n261 = property on="Test Slider" class="Slide (strict)"("Visible"=w420) -> ()  [unwired: 2 in, 2 out]
        n262 = property on="On/Off" class="Bool (strict)"("Visible"=w420) -> ()  [unwired: 2 in, 2 out]
        n263 = property on="Rev/Fwd" class="Clust (strict)"("Visible"=w420) -> ()  [unwired: 2 in, 2 out]
        n264 = property on="Test Ring" class="Ring (strict)"("Visible"=w420) -> ()  [unwired: 2 in, 2 out]
      }
      event "Select Auto": Mouse Enter {
        # "Populate the combo box with the list of autonomous options"
        n265 = event-data() -> ()  [unwired: 1 in, 1 out]
        n266 = call <vilib>:"NT Read String Array.vi"("Name"="Auto List") -> ("String Array"=w427:string[])  [unwired: 9 in, 1 out]
        n267 = property on="Select Auto" class="CmbBox"("Strings[]"=w427) -> ()  [unwired: 2 in, 2 out]
      }
      event "Select Auto": Value Change {
        # "User modified the Auto Selection. Write to NT variable so robot knows."
        n268 = event-data() -> ("NewVal"=w430:string)  [unwired: 1 in]
        n269 = call <vilib>:"NT Write String.vi"("String"=w430, "Name"="Auto Selector") -> ()  [unwired: 9 in, 1 out]
      }
      event "Command Selection": Value Change {
        # "Get the params and show in table"
        n270 = event-data() -> ("NewVal"=w436:i32)  [unwired: 1 in]
        n271 = property on="Command Selection" class="MCListbox (strict)"() -> ("ItemNames"=w434:string[][])  [unwired: 2 in, 2 out]
        n272 = call <vilib>:"WPI_DashboardUpdate Command Params.vi"("NewVal"=w436, "Commands"=w434, "Param Tbl"=w435) -> ()  [unwired: 8 in, 1 out]
      }
      event "Execute Command": Value Change {
        # "Started one, Unique ID holds\nresponse"
        n273 = event-data() -> ()  [unwired: 1 in, 1 out]
        n274 = property on="Command Selection" class="MCListbox (strict)"() -> ("ItemNames"=w447:string[][])  [unwired: 2 in, 2 out]
        n275 = Index Array(array=w447, index (row)="Command Selection", index (col)=0) -> (element=w445:string)
        n276 = call <vilib>:"Invoke Commands.vi"("Command Params"="Command Params", "Function Name"=w445) -> ("Params"=w441:u8, "Started"=w440:bool)  [unwired: 7 in, 1 out]
        n277 = Array Subset(array="Command Params", length (row)=w441) -> (w442:string[][])  [unwired: 3 in]
        n278 = Select(t="Executing" ("Cmd Status"), s=w440, f="" ("Cmd Status")) -> (s? t:f=→"Cmd Status":string)
      }
      event "Command Selection": Double Click {
        n279 = event-data() -> ("Row"=w455:i32)  [unwired: 1 in]
        n280 = property on="Command Selection" class="MCListbox (strict)"() -> ("ItemNames"=w458:string[][])  [unwired: 2 in, 2 out]
        n281 = local read "Command Params"() -> (w454:string[][])
        n282 = Index Array(array=w458, index (row)=w455, index (col)=0) -> (element=w456:string)
        n283 = call <vilib>:"Invoke Commands.vi"("Command Params"=w454, "Function Name"=w456) -> ("Params"=w453:u8, "Started"=w448:bool)  [unwired: 7 in, 1 out]
        n284 = Array Subset(array=w454, length (row)=w453) -> (w452:string[][])  [unwired: 3 in]
        n285 = Select(t="Executing" ("Cmd Status"), s=w448, f="" ("Cmd Status")) -> (s? t:f=w449:string)
        n286 = local write "Cmd Status"(w449) -> ()
      }
      event "CheckList": Double Click {
        # "Shift clears all"
        # "Update symbols on the listbox"
        n287 = event-data() -> ("PlatMods.Shift"=w460:bool, "Row"=w462:i32)  [unwired: 1 in]
        n288 = case shown="True" w460 {
          tunnel: w462 -> [w466 _]
          tunnel: 1 -> [w465 _]
          frame False {
            n289 = property on="CheckList" class="LstBox (strict)"() -> ("Item Symbols"=w464:i32[])  [unwired: 2 in, 2 out]
            n290 = Replace Array Subset(array=w464, new element=w465, index=w466) -> (w463:i32[])
            n291 = property on="CheckList" class="LstBox (strict)"("Item Symbols"=w463) -> ()  [unwired: 2 in, 2 out]
          }
          frame True {
            w467 = 0 ("Top Row")
            n292 = property on="CheckList" class="LstBox (strict)"() -> ("Number of Rows"=w469:u32)  [unwired: 2 in, 2 out]
            n293 = Initialize Array(0, w469) -> (w468:i32[])
            n294 = property on="CheckList" class="LstBox (strict)"("Top Row"=w467, "Value"=w467, "Item Symbols"=w468) -> ()  [unwired: 2 in, 2 out]
          }
        }
      }
      event "CheckList": Key Down {
        # "Update symbols on the listbox\nLeft and right keys check and uncheck"
        n295 = event-data() -> ("VKey"=w473:T22)  [unwired: 1 in]
        n296 = case shown="\"Left\", \"Right\"" w473 {
          selector: w473 -> [w478 _]
          tunnel: eventvkey."Left" ("VKey") -> [w476 _]
          frame "Left", "Right" {
            n297 = Equal?(x=w476, y=w478) -> (x = y?=w477:bool)
            n298 = Select(t=0, s=w477, f=1) -> (s? t:f=w479:i32)
            n299 = property on="CheckList" class="LstBox (strict)"() -> ("Item Symbols"=w482:i32[])  [unwired: 2 in, 2 out]
            n300 = Replace Array Subset(array=w482, new element=w479, index="CheckList") -> (w481:i32[])
            n301 = property on="CheckList" class="LstBox (strict)"("Item Symbols"=w481) -> ()  [unwired: 2 in, 2 out]
          }
          frame Default {
          }
        }
      }
      event "Motor.Enable": Value Change {
        # "When the test mode otor enable helper is set, update that\ntree row item's value"
        n302 = event-data() -> ("NewVal"=w488:bool)  [unwired: 1 in]
        n303 = Unbundle("Motor") -> ("Value"=w487:dbl)  [unwired: 1 out]
        n304 = Select(t=w487, s=w488, f=0.0) -> (s? t:f=w485:dbl)
        n305 = call <vilib>:"NT Write Number.vi"("Numeric"=w485, "Name"=w484) -> ()  [unwired: 9 in, 1 out]
      }
      event "Test Slider": Value Change {
        # "When the test mode slider helper is set, update that\ntree row item's value"
        n306 = event-data() -> ("NewVal"=w491:dbl)  [unwired: 1 in]
        n307 = call <vilib>:"NT Write Number.vi"("Numeric"=w491, "Name"=w492) -> ()  [unwired: 9 in, 1 out]
      }
      event "On/Off": Value Change {
        # "When the test mode on/off helper value is set, update that\ntree row item's value"
        n308 = event-data() -> ("NewVal"=w496:bool)  [unwired: 1 in]
        n309 = Boolean To (0,1)(Boolean=w496) -> (0, 1=w495:i16)
        n310 = call <vilib>:"NT Write Number.vi"("Numeric"=w495, "Name"=w494) -> ()  [unwired: 9 in, 1 out]
      }
      event "Rev/Fwd": Value Change {
        # "When the test mode helper value for relays is set, update that\ntree row item's value"
        n311 = event-data() -> ("NewVal.Forward"=w504:bool, "NewVal.Reverse"=w503:bool)  [unwired: 1 in]
        n312 = Boolean To (0,1)(Boolean=w504) -> (0, 1=w500:i16)
        n313 = Boolean To (0,1)(Boolean=w503) -> (0, 1=w502:i16)
        n314 = Negate(x=w502) -> (-x=w501:i16)
        n315 = Add(x=w500, y=w501) -> (x+y=w499:i16)
        n316 = call <vilib>:"NT Write Number.vi"("Numeric"=w499, "Name"=w498) -> ()  [unwired: 9 in, 1 out]
      }
      event "Test Ring": Value Change {
        # "When a test mode helper value is selected from the ring,\nset the tree item's variable to the string value"
        n317 = event-data() -> ("NewVal"=w508:u16)  [unwired: 1 in]
        n318 = property on="Test Ring" class="Ring (strict)"() -> ("Strings []"=w509:string[])  [unwired: 2 in, 2 out]
        n319 = Index Array(array=w509, index=w508) -> (element=w507:string)
        n320 = call <vilib>:"NT Write String.vi"("String"=w507, "Name"=w506) -> ()  [unwired: 9 in, 1 out]
      }
      event "Rec Mode": Value Change {
        # "Update globals for recording mode and path to read log from.\nClear when logging and let NetworkTables set path for vision to\nuse."
        n321 = event-data() -> ("NewVal"=w520:enum32{"Stop", "Record", "Playback"})  [unwired: 1 in]
        n322 = global write "WPI_DashboardLogging Global.vi" "Logging Filename"(path "") -> ()
        n323 = global write "WPI_DashboardLogging Global.vi" "Recording"(w520) -> ()
        n324 = case shown="\"Playback\"" w520 {
          tunnel: w519 -> [_ w522 w531]
          tunnel: [_ _ w530] -> w517
          tunnel: [_ _ w529] -> _
          tunnel: w515 -> [_ _ w527]
          tunnel: cluster{i32, i32} {-250, 170} -> [_ _ w526]
          tunnel: [_ _ T23 {"Image Size"=TRUE, "Image Type"=TRUE, "Pixel Value"=TRUE, "ROI Information"=TRUE, "Zoom Factor"=FALSE} ("Image Information Shown:All Elements")] -> w510
          tunnel: [_ _ TRUE ("Zoom Factor")] -> w511
          tunnel: w513 -> [_ _ w523]
          frame Default {
          }
          frame "Stop", "Record" {
            # "Place Window too"
            n325 = invoke class="VI" method="FP.Close"(reference=w522) -> (reference out=w521:refnum<vi>)  [unwired: 2 in, 2 out]
            n326 = invoke class="VI" method="Abort VI"(reference=w521) -> ()  [unwired: 2 in, 3 out]
          }
          frame "Playback" {
            n327 = call "Open Playback Panel.vi"("Offset"=w526, "DB VI Ref"=w527, "Playback in"=w531) -> ("Playback out"=w528:refnum<vi>)  [unwired: 8 in]
            n328 = register-events(w528, w523) -> (reference out=w530:refnum<event-registration>, error out=w529:errorcluster)  [unwired: 2 in]
          }
        }
        n329 = property on="Camera Image Right" class="ImageControl"("Image Information Shown"=w510, "Image Information Visible"=w511) -> ()  [unwired: 2 in, 2 out]
        n330 = property on="Camera Image" class="ImageControl"("Image Information Shown"=w510, "Image Information Visible"=w511) -> ()  [unwired: 2 in, 2 out]
        n331 = call <vilib>:"WPI_DashboardNT Log FieldName Cache.vi"("Operation"=enum16{"Lookup/Add", "Index", "Clear"}."Clear") -> ()  [unwired: 8 in, 3 out]
      }
      event Panel Close {
        w533 = enum32{"Stop", "Record", "Playback"}."Stop" ("Rec Mode")
        # "Playback window has been closed, abort"
        n332 = event-data() -> ()  [unwired: 1 in, 4 out]
        n333 = local write "Rec Mode"(w533) -> ()
        n334 = global write "WPI_DashboardLogging Global.vi" "Recording"(w533) -> ()
      }
      event Panel Close {
        # "Abort playback window and ourself"
        n335 = event-data() -> ()  [unwired: 1 in, 4 out]
        n336 = invoke class="VI" method="FP.Close"(reference=w537) -> (reference out=w536:refnum<vi>)  [unwired: 2 in, 2 out]
        n337 = invoke class="VI" method="Abort VI"(reference=w536) -> (error out=w535:errorcluster)  [unwired: 2 in, 2 out]
        n338 = invoke class="VI" method="Abort VI"(error in=w535) -> ()  [unwired: 2 in, 3 out]
      }
      event User Event {
        n339 = event-data() -> ("IDs"=w544:cluster{"RPC field ID":u16, "Unique ID":u16}, "String"=w543:string)  [unwired: 1 in]
        n340 = Bundle("IDs"=w544, "String"=w543) -> (w542:T9)  [unwired: 1 in]
        n341 = call <vilib>:"Retrieve RPC Response.vi"("RPC Response"=w542) -> ("Output"=w540:string[][])  [unwired: 10 in]
        n342 = Build Array (concatenate)(w538, w540) -> (w539:string[][])
        n343 = local write "Command Params"(w539) -> ()
        n344 = local write "Cmd Status"("" ("Cmd Status")) -> ()
      }
      event "Tree": Double Click {
        n345 = event-data() -> ("PlatMods"=w550:T26, "Tag"=w547:string)  [unwired: 1 in]
        n346 = Unbundle(w550) -> ("Shift"=w549:bool)  [unwired: 4 out]
        n347 = String Subset(string=w547, length (rest)=1 ("length (rest)")) -> (substring=w546:string)  [unwired: 1 in]
        n348 = Not(x=w549) -> (.not. x?=w548:bool)
        n349 = case shown="\"/\"" w546 {
          tunnel: w547 -> [_ w553]
          tunnel: w548 -> [_ w552]
          frame Default {
          }
          frame "/" {
            n350 = call <vilib>:"NT Update Persistence.vi"("Persistence"=w552, "Name"=w553) -> ()  [unwired: 9 in, 1 out]
          }
        }
      }
    }
  }
  n351 = while {
    tunnel: w65 -> [w555]
    i -> [w558]
    stop <- FALSE stop-if-true
    n352 = Wait (ms)(milliseconds to wait=u32 100) -> ()  [unwired: 1 out]
    n353 = case shown="\"Playback\"" "Rec Mode" {
      tunnel: w558 -> [_ _ w573]
      tunnel: [u32 2829099 ("Base Color") u32 11141120 ("Target Color") w562] -> w554
      frame "Stop", Default {
        # "Reset the color, extra updates don't cost much"
      }
      frame "Record" {
      }
      frame "Playback" {
        # "Playback"
        n354 = Quotient & Remainder(x=w573, y=u32 50 ("milliseconds to wait")) -> (x-y*floor(x/y)=w569:u32)  [unwired: 1 out]
        n355 = Divide(x=w569, y=u32 50 ("milliseconds to wait")) -> (x/y=w566:dbl)
        n356 = Multiply(x=6.283185307179586, y=w566) -> (x*y=w571:dbl)
        n357 = Sine(x=w571) -> (sin(x)=w570:dbl)
        n358 = Absolute Value(x=w570) -> (abs(x)=w563:dbl)
        n359 = call "Interpolate RGB Color.vi"("Proportion"=w563, "Target Color"=u32 30976, "Base Color"=u32 2829099) -> ("Result Color"=w562:u32)  [unwired: 8 in]
      }
    }
    n360 = property class="Pane"(reference=w555, "PaneColor"=w554) -> ()  [unwired: 1 in, 2 out]
  }
  n361 = local write "Dashboard Tab"(T2."Drive" ("Dashboard Tab")) -> ()
  n362 = property on="On/Off" class="Bool (strict)"("Visible"=w36) -> ()  [unwired: 2 in, 2 out]
  n363 = property on="Motor" class="Clust (strict)"("Visible"=w36) -> ()  [unwired: 2 in, 2 out]
  n364 = property on="Progress" class="Clust (strict)"("Visible"=w36) -> ()  [unwired: 2 in, 2 out]
  n365 = property on="Test Ring" class="Ring (strict)"("Visible"=w36) -> ()  [unwired: 2 in, 2 out]
  n366 = property on="Rev/Fwd" class="Clust (strict)"("Visible"=w36) -> ()  [unwired: 2 in, 2 out]
  n367 = while {
    tunnel: u16 1741 ("timeout ms (25000)") -> [w575]
    stop <- FALSE stop-if-true
    n368 = TCP Create Listener(10:w575) -> (0:w574:errorcluster, 3:w576:refnum<k5>)  [unwired: 4 in, 1 out]
    n369 = case shown="No Error" w574 {
      selector: w574 -> [w578 _]
      tunnel: w576 -> [w579 _]
      frame No Error {
        n370 = while {
          tunnel: w579 -> [w582]
          tunnel: w578 -> [w581]
          stop <- FALSE stop-if-true
          n371 = TCP Wait On Listener(8:w581, 11:w582) -> (0:w583:errorcluster, 4:w584:refnum<k5>)  [unwired: 2 in, 3 out]
          n372 = local write "TCP"(w584) -> ()
          n373 = case shown="No Error" w583 {
            frame No Error {
            }
            frame Error {
              n374 = Wait (ms)(milliseconds to wait=u32 1000) -> ()  [unwired: 1 out]
            }
          }
        }
      }
      frame Error {
        n375 = Wait (ms)(milliseconds to wait=u32 1000) -> ()  [unwired: 1 out]
      }
    }
  }
  n376 = local write "Command Selection"(u16 0 ("milliseconds to wait")) -> ()
  n377 = local write "Command Params"(string[][] [] ("Command Params")) -> ()
  n378 = global write "WPI_DashboardLogging Global.vi" "Recording"(w59) -> ()
  n379 = local write "Rec Mode"(w59) -> ()
  n380 = call <vilib>:"NT Write String.vi"("String"="Select Auto", "Name"="Auto Selector") -> ()  [unwired: 9 in, 1 out]
